vi "DSF.Shared.Configuration.Transfer.Get Byte Order.vi"(11 "Transfer Configuration in":refnum<class "DSF.Shared.Configuration.Transfer.lvclass">) -> (2 "byte order":T1, 3 "Transfer Configuration out":refnum<class "DSF.Shared.Configuration.Transfer.lvclass">)   [LabVIEW 2017, in "DSF.Engine.lvlib" / "DSF.Shared.Configuration.Transfer.lvclass"]
uses:
  DSF.Shared.Configuration.Transfer.lvclass
  Typedefs/DSF.Shared.Typedefs.Byte Order.ctl
  DSF.Shared.Configuration.Transfer.lvclass/DSF.Shared.Configuration.Transfer.ctl
  DSF.Engine.lvlib
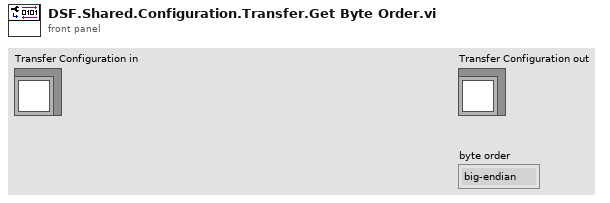
[diagram p1: front panel]
types:
  T1 = typedef "DSF.Engine.lvlib/DSF.Shared.Typedefs.Byte Order.ctl" = enum8{"big-endian", "little-endian"}
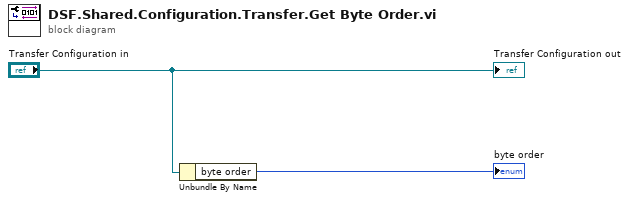
[diagram p0: block diagram]
diagram:
  n1 = Unbundle By Name("Transfer Configuration in") -> ("byte order"=→"byte order":T1)
  "Transfer Configuration out" <- "Transfer Configuration in"
